vi "Read Force Table Settings.vi"(8 "error in (no error)":errorcluster, 11 "Boot Loader in":refnum<class "Boot Loader.lvclass">) -> (0 "error out":errorcluster, 2 "Force Table Settings":T1 {"Entries"."Force Set Points"."Axial Force" format="%.4f"; "Entries"."Force Set Points"."Lateral Force" format="%.4f"}, 3 "Boot Loader out":refnum<class "Boot Loader.lvclass">)   [LabVIEW 2016, in "Boot Loader.lvclass"]
uses:
  Boot Loader.lvclass
  Typedefs/ForceTableSettings.ctl
  Typedefs/ForceTableEntry.ctl
  Typedefs/ForcePair.ctl
  Settings/Settings.lvclass
  Typedefs/FAMT Typedefs.lvlib
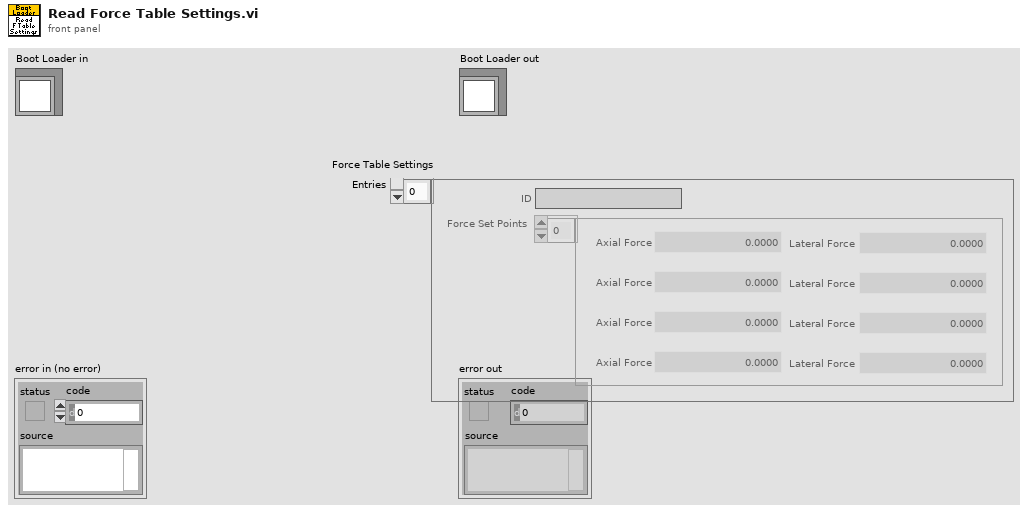
[diagram p1: front panel]
types:
  T1 = typedef "FAMT Typedefs.lvlib/ForceTableSettings.ctl" = cluster{"Entries":T2[]}
  T2 = typedef "FAMT Typedefs.lvlib/ForceTableEntry.ctl" = cluster{"ID":string, "Force Set Points":T3[]}
  T3 = typedef "FAMT Typedefs.lvlib/ForcePair.ctl" = cluster{"Axial Force":dbl, "Lateral Force":dbl}
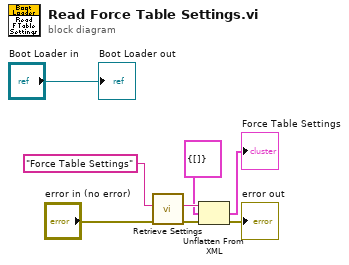
[diagram p0: block diagram]
diagram:
  n1 = call "Retrieve Settings.vi"("error in (no error)"="error in (no error)", "configName"="Force Table Settings") -> ("error out"=w4:errorcluster, "xmlConfig"=w7:string)  [unwired: 7 in, 1 out]
  n2 = Unflatten From XML(xml string=w7, type=T1 {"Entries"=[]} ("Force Table Settings"), error in (no error)=w4) -> (value=→"Force Table Settings":T1, error out=→"error out":errorcluster)
  "Boot Loader out" <- "Boot Loader in"
